vi "DeInit Done.vi"(8 "error in (no error)":errorcluster, 9 "Initialized":bool, 10 "InstrumentData":T1, 11 "SLM_Controller in":refnum<class "SLM_Controller.lvclass">) -> (0 "error out":errorcluster, 3 "SLM_Controller out":refnum<class "SLM_Controller.lvclass">)   [LabVIEW 2023, in "SLM_Controller.lvlib" / "SLM_Controller.lvclass"]
uses:
  typedefs/InstrumentData.ctl
  typedefs/instrumentType.ctl
  SLM_Controller.lvclass
  SLM_Controller.lvclass/SLM_Controller.ctl
  typedefs/typedefs.lvlib
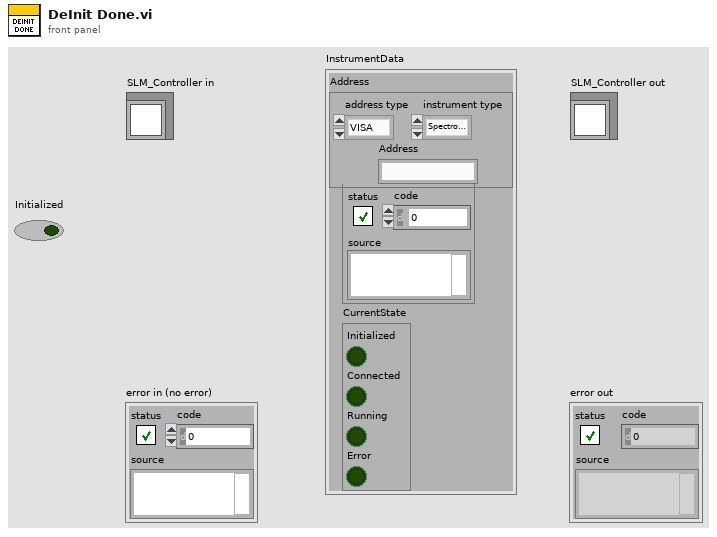
[diagram p1: front panel]
types:
  T1 = typedef "typedefs.lvlib/InstrumentData.ctl" = cluster{"Instr Error":errorcluster, "Address":cluster{"address type":enum16{"VISA", "Index"}, "Address":string, "instrument type":T2}, "CurrentState":cluster{"Initialized":bool, "Connected":bool, "Running":bool, "Error":bool}}
  T2 = typedef "typedefs.lvlib/instrumentType.ctl" = enum16{"Spectrometer", "Camera", "Stepper", "Piezo"}
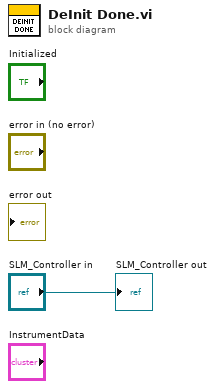
[diagram p0: block diagram]
diagram:
  "SLM_Controller out" <- "SLM_Controller in"
